vi "09_another_example.vi"() -> ()   [LabVIEW 2018, in "LV2Julia_examples.lvlib"]
uses:
  LV2Julia_examples.lvlib
  LV2Julia_core/VIs/Server or client state.ctl
  LV2Julia_core/VIs/detailed error info.ctl
  LV2Julia_core/VIs/StackFrame.ctl
  simple examples functions.ctl
  LV2Julia_core/VIs/Commands.ctl
  63b50369-e720-4ad2-b7fe-b63add1d9180.vi
  edf81fa3-46bf-427f-9605-85b461656974.vi
  29886417-d43f-41fb-9c0c-469db3f8c96d.vi
  3fe35f36-217a-40a5-a789-8326c52a1f5c.vi
  8d86b089-302c-401c-ae82-d9ebdf0ff266.vi
  35a44a82-786b-41ea-be73-9a4468e4df9d.vi
  a43e0667-dcfc-466a-94c9-f7da2d4fd36f.vi
  <vilib>/Utility/High Resolution Relative Seconds.vi
  edf81fa3-46bf-427f-9605-85b461656974.vi/ed560bc2-c7a5-459b-9b5d-c09f4150f87a.vi
  29886417-d43f-41fb-9c0c-469db3f8c96d.vi/351cf3e2-3c27-4899-8ca9-cb74734acfc8.vi
  3fe35f36-217a-40a5-a789-8326c52a1f5c.vi/3d491d8d-1e21-4aec-9a68-d7bbb94dfa6b.vi
  35a44a82-786b-41ea-be73-9a4468e4df9d.vi/70e9cb77-3a98-433e-ba66-4dcec83fe426.vi
  35a44a82-786b-41ea-be73-9a4468e4df9d.vi/c7757579-5117-4a7e-a803-a4a1d792155f.vi
  edf81fa3-46bf-427f-9605-85b461656974.vi/ed560bc2-c7a5-459b-9b5d-c09f4150f87a.vi/acba61d8-f5e3-4002-bc70-34f15e56434e.vi
  29886417-d43f-41fb-9c0c-469db3f8c96d.vi/351cf3e2-3c27-4899-8ca9-cb74734acfc8.vi/26bd0686-ce58-4dc2-9cfb-ec11559fc1fa.vi
  29886417-d43f-41fb-9c0c-469db3f8c96d.vi/351cf3e2-3c27-4899-8ca9-cb74734acfc8.vi/31514e23-2cd5-4295-b47a-a1ad325a4df0.vi
  29886417-d43f-41fb-9c0c-469db3f8c96d.vi/351cf3e2-3c27-4899-8ca9-cb74734acfc8.vi/3d30d75b-34ec-4e52-a519-b86950648cc6.vi
  3fe35f36-217a-40a5-a789-8326c52a1f5c.vi/3d491d8d-1e21-4aec-9a68-d7bbb94dfa6b.vi/5fb8a6ea-f43c-4306-9aef-f7be33a28f7f.vi
  3fe35f36-217a-40a5-a789-8326c52a1f5c.vi/3d491d8d-1e21-4aec-9a68-d7bbb94dfa6b.vi/dfcd26d4-3f06-4489-82d4-95ea86395353.vi
  3fe35f36-217a-40a5-a789-8326c52a1f5c.vi/3d491d8d-1e21-4aec-9a68-d7bbb94dfa6b.vi/9b688aa8-4353-46ee-ad38-c3c6feb92501.vi
  35a44a82-786b-41ea-be73-9a4468e4df9d.vi/70e9cb77-3a98-433e-ba66-4dcec83fe426.vi/97f29e4c-2cc7-47ea-9755-65b879169f6c.vi
  35a44a82-786b-41ea-be73-9a4468e4df9d.vi/70e9cb77-3a98-433e-ba66-4dcec83fe426.vi/9acd3ce5-a096-44ea-970d-7ed2f22121f9.vi
  edf81fa3-46bf-427f-9605-85b461656974.vi/ed560bc2-c7a5-459b-9b5d-c09f4150f87a.vi/acba61d8-f5e3-4002-bc70-34f15e56434e.vi/0e04b98d-ee84-41a3-96e8-138e19c14a1d.vi
  35a44a82-786b-41ea-be73-9a4468e4df9d.vi/70e9cb77-3a98-433e-ba66-4dcec83fe426.vi/97f29e4c-2cc7-47ea-9755-65b879169f6c.vi/a4bd5a91-b8fb-45c2-8725-513a162f3679.vi
  LV2Julia_core/VIs/jl-scripts path.vi
  LV2Julia_core/VIs/check ID validity.vi
  LV2Julia_core/VIs/bindata_descr to JSON.vi
  LV2Julia_core/VIs/check cluster field names.vi
  LV2Julia_core/VIs/concat JSON.vi
  LV2Julia_core/VIs/build request.vi
  LV2Julia_core/VIs/Parse server response.vi
  LV2Julia_core/VIs/log jl exceptions.vi
  <vilib>/Utility/error.llb/Error Cluster From Error Code.vi
  LV2Julia_core/LV2Julia_core.lvlib
  <vilib>/measure/NI_MABase.lvlib
panel:
  out "ZMQ timeout":bool
  out "Julia script file path":path
  out "temporary script path":path
  out "Jl Server state":T1
  in  "execution control pages":enum32{"Start", "go - test"}(tab)
  in  "go":bool caption="go (Julia Server started externally)"
  in  "Start with Julia":bool caption="Start Julia Server and go"
  in  "ZMQ endpoint":string="tcp://127.0.0.1:5555"
  in  "p":dbl=1.0
  in  "fn":T2 caption="select function at Server" items=["arr_amplitude", "arr_length", "arr_mean", "arr_median", "arr_rms", "vec_amplify", "vec_attenuate", "vec_power"]
  in  "trim @ begin":dbl min=0.0 max=100.0 step=1.0 format="%#.1f%%"
  in  "trim @ end":dbl min=0.0 max=200.0 step=1.0 format="%#.1f%%"
  in  "Group":T3(tab)
  out "Server response":dbl
  out "data received plot":dbl[](graph)
  out "data received":dbl[](array[numeric]) format="%.3f"
  out "RMS":dbl
  out "detailed error info":T4
  out "current error":errorcluster
  out "final error":errorcluster
  out "short err code":u8
  in  "tones":T6(array[cluster])=[{"frequency"=10.0, "amplitude"=1.0, "phase"=0.0}, {"frequency"=20.0, "amplitude"=0.1, "phase"=0.0}] {"phase" format="%.2p"; "amplitude" format="%0.2p"; "frequency" format="%0.2p"}
  in  "noise (rms)":dbl=0.1 format="%.2p"
  in  "offset":dbl format="%.2p"
  in  "sampling info":cluster{"Fs":dbl, "#s":dbl}={"Fs"=1000.0, "#s"=1000.0} {"Fs" format="%.2p"}
  in  "next":bool
  out "data sent to server":dbl[](graph)
  out "data sent":dbl[](array[numeric]) format="%.3f"
  out "function name":string
  in  "stop this VI only":bool
  in  "stop both this VI and Julia Server":bool
  out "call duration (ms)":dbl format="%#.2f"
  # "tcp://127.0.0.1:5555 \nfor local Julia Server\n\nFor a Julia Server running on a separate computer,  you probably must use an IPv4 address in numeric form (not a DNS name) - see https://stackoverflow.com/questions/6024003/why-doesnt-zeromq-work-on-localhost.\n\nThis control only used if Julia Server is not being started by this VI."
  # "generate sample array"
  # "function and parameter"
  # "enter a negative or a large positive value to cause an exception"
  # "data returned by server"
  # "data sent to server"
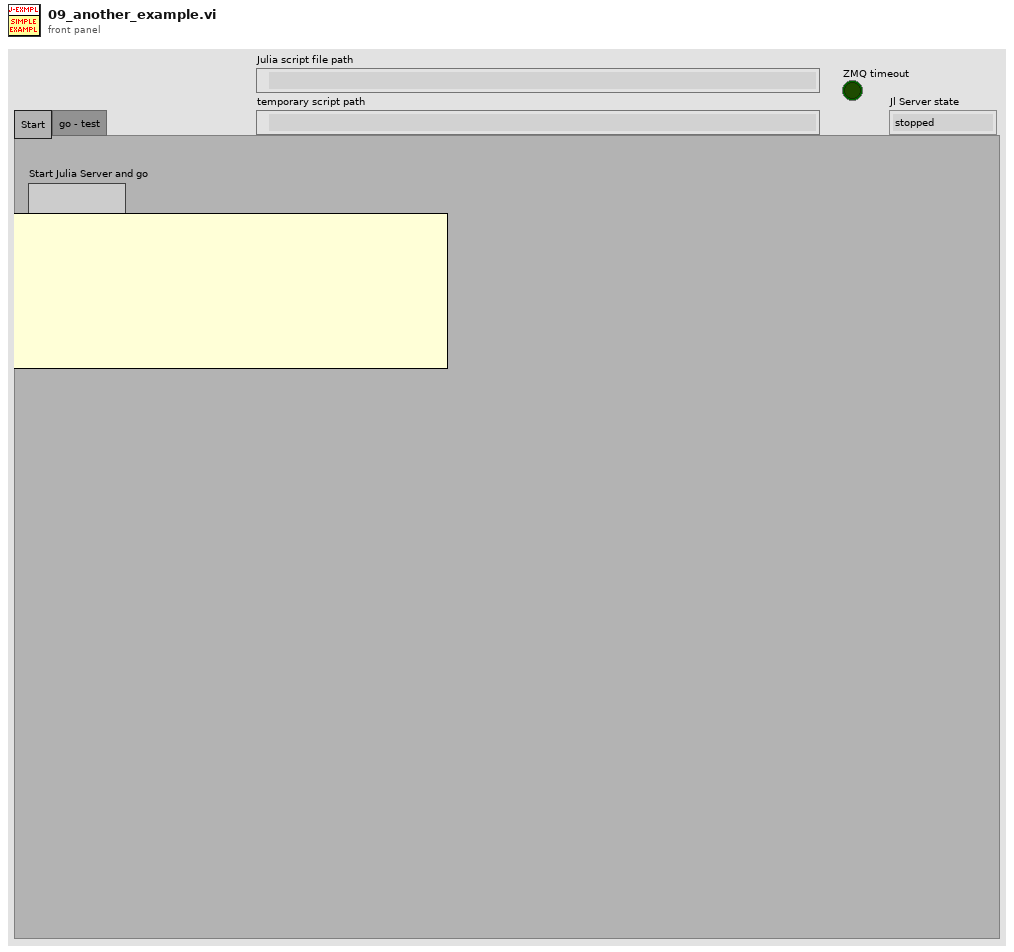
[diagram p1: front panel]
types:
  T1 = typedef "LV2Julia_core.lvlib/Server or client state.ctl" = enum16{"stopped", "running", "unknown"}
  T2 = typedef "LV2Julia_examples.lvlib/simple examples functions.ctl" = u16
  T3 = enum32{"fns returning scalar", "fns returning vector", "error"}
  T4 = typedef "LV2Julia_core.lvlib/detailed error info.ctl" = cluster{"exception_or_info":string, "trace":T5[]}
  T5 = typedef "LV2Julia_core.lvlib/StackFrame.ctl" = cluster{"frame_summary":string, "func":string, "linfo":string, "file":string, "line":i32, "pointer":u64, "from_c":bool, "inlined":bool}
  T6 = cluster{"frequency":dbl, "amplitude":dbl, "phase":dbl}[]
  T7 = typedef "LV2Julia_core.lvlib/Commands.ctl" = enum16{"Start Jl-server & Init LV-client", "Send request & Get response ", "Stop Jl-server & Cleanup LV-client", "Cleanup LV-client", "Start Jl-server", "Stop Jl-server", "Init LV-Client", "Cleanup LV-Client", "(not allowed)", "Set LV Client state", "Set Jl Server state", "set ZMQ timeout", "read ZMQ timeout", "read-out state"}
  T8 = enum8{"Enabled", "Disabled", "Disabled and Grayed Out"}
  T9 = typedef "LV2Julia_core.lvlib/Bindata&description.ctl" = cluster{"bindata_descr":T10[], "bindata":u8[]}
  T10 = typedef "LV2Julia_core.lvlib/Bindata description.ctl" = cluster{"nofbytes":i32, "numtype":string, "start":i32, "arrdims":i32[], "kwarg_name":string, "category":string}
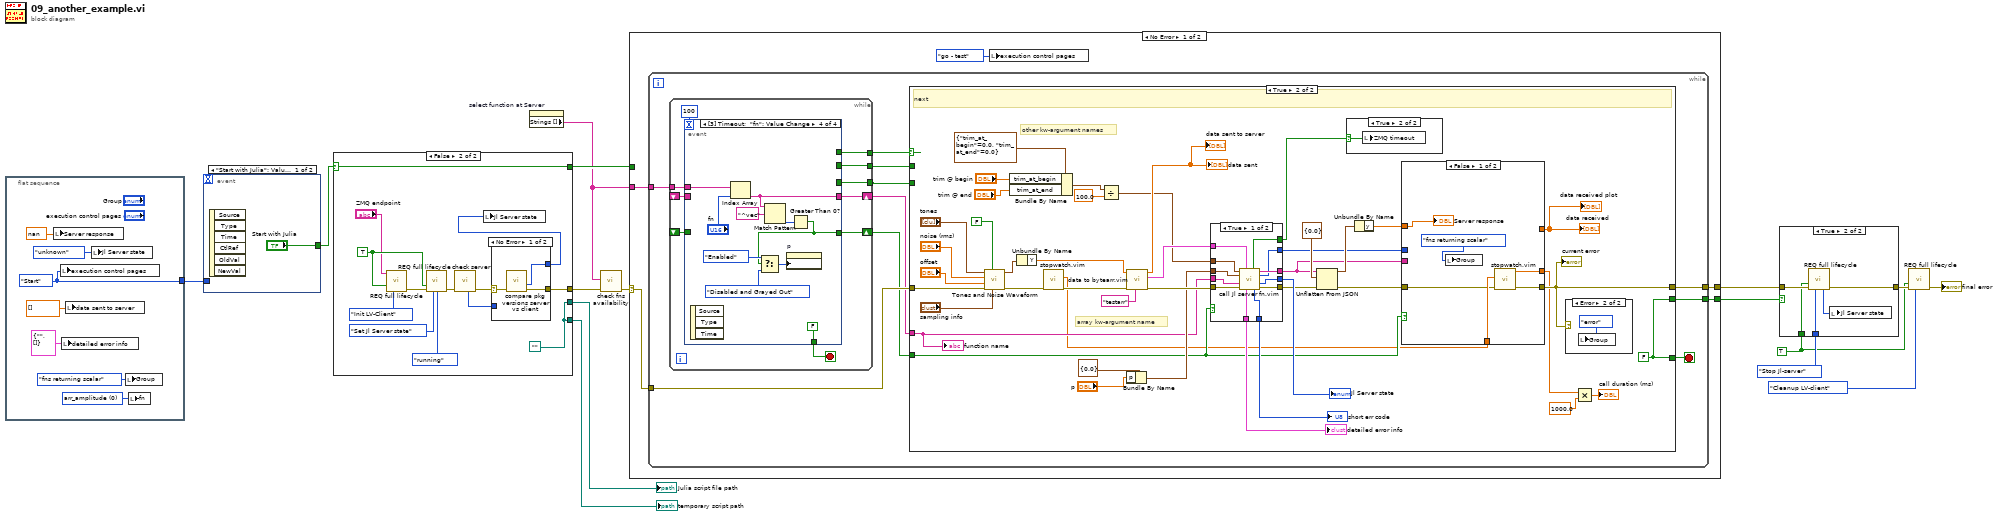
[diagram p0: block diagram]
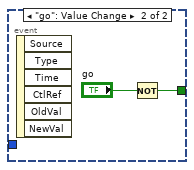
[diagram p2: hidden frame]
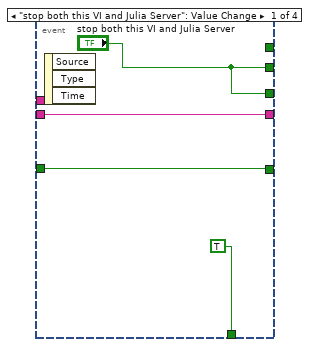
[diagram p3: hidden frame]
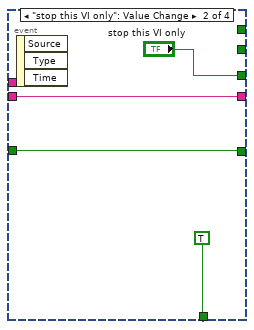
[diagram p4: hidden frame]
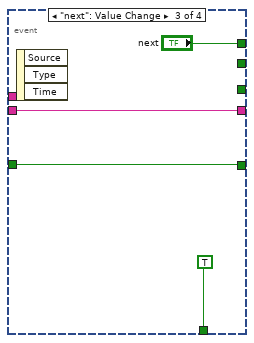
[diagram p5: hidden frame]
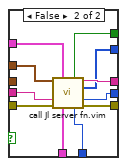
[diagram p7: hidden frame]
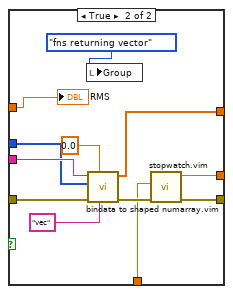
[diagram p9: hidden frame]
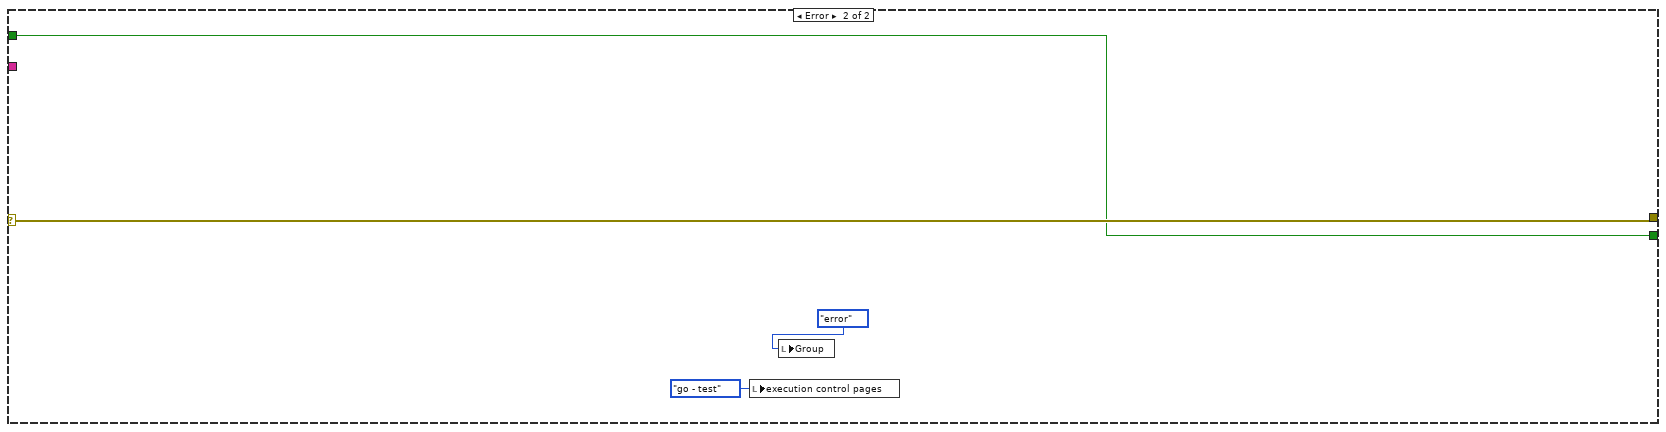
[diagram p11: hidden frame]
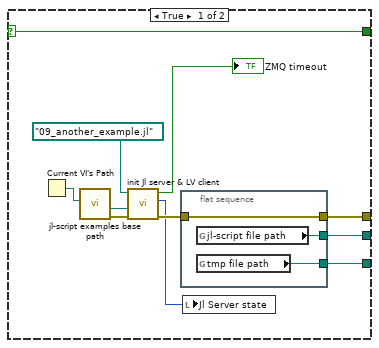
[diagram p12: hidden frame]
diagram:
  w10 = TRUE ("Force command")
  n1 = flat-sequence {
    tunnel: [w22] -> w6
    frame #0 {
      w16 = T2 0 items=["arr_amplitude", "arr_length", "arr_mean", "arr_median", "arr_rms", "vec_amplify", "vec_attenuate", "vec_power"] ("fn")
      w22 = enum32{"Start", "go - test", "finish"}."Start" ("execution control pages")
      n2 = local write "Server response"(nan ("Server response")) -> ()
      n3 = local write "execution control pages"(w22) -> ()
      n4 = local write "detailed error info"(T4 {"exception_or_info"="", "trace"=[]} ("detailed error info")) -> ()
      n5 = local write "data sent to server"(dbl[] []) -> ()
      n6 = local write "Jl Server state"(Server_or_client_state."unknown" ("Jl Server state out")) -> ()
      n7 = local write "Group"(T3."fns returning scalar" ("Group")) -> ()
      n8 = local write "fn"(w16) -> ()
    }
  }
  n9 = event shown="[0] \"Start with Julia\": Value Change" {
    selector: _ -> [_ _]
    dyn-events: _ -> [_ _]
    timeout: _ -> [_ _]
    tunnel: ["Start with Julia" w24] -> w8
    tunnel: w6 -> [_ _]
    event "Start with Julia": Value Change {
      n10 = event-data() -> ()  [unwired: 1 in, 6 out]
    }
    event "go": Value Change {
      n11 = event-data() -> ()  [unwired: 1 in, 6 out]
      n12 = Not(x="go") -> (.not. x?=w24:bool)
    }
  }
  n13 = case shown="False" w8 {
    selector: w8 -> [w36 w48]
    tunnel: [w35 w42] -> w5
    tunnel: [w36 w48] -> w7
    tunnel: [w34 w45] -> w1
    tunnel: [w33 w45] -> w2
    frame True {
      n14 = Current VI's Path() -> (path=w28:path)
      n15 = call "jl-script examples base path.vi"("calling example VI path"=w28) -> ("error out"=w27:errorcluster, "jl-script-examples base path"=w26:path)  [unwired: 9 in]
      n16 = call "init Jl server & LV client.vi"("error in (no error)"=w27, "Base path (not a path)"=w26, "Julia user functions script"=path "09_another_example.jl") -> ("error out"=w30:errorcluster, "Jl Server state out"=w29:T1, "timeout?"=→"ZMQ timeout":bool)  [unwired: 6 in]
      n17 = flat-sequence {
        tunnel: [w39] -> w35
        tunnel: w30 -> [w39]
        tunnel: [w38] -> w34
        tunnel: [w37] -> w33
        frame #0 {
          n18 = global read "jl-scripts path.vi" "jl-script file path"() -> (w38:path)
          n19 = global read "jl-scripts path.vi" "tmp file path"() -> (w37:path)
        }
      }
      n20 = local write "Jl Server state"(w29) -> ()
    }
    frame False {
      w45 = path ""
      w50 = TRUE ("Force command")
      n21 = call "REQ full lifecycle.vi"("ZMQ endpoint"="ZMQ endpoint", "Force command"=w50, "command"=Commands."Init LV-Client") -> ("error out"=w47:errorcluster)  [unwired: 6 in, 6 out]
      n22 = call "REQ full lifecycle.vi"("Force command"=w50, "error in"=w47, "command"=Commands."Set Jl Server state", "Jl Server state in"=Server_or_client_state."running") -> ("error out"=w46:errorcluster)  [unwired: 5 in, 6 out]
      n23 = call "check server.vi"("error in"=w46) -> ("error out"=w43:errorcluster, "Jl Server state out"=w41:T1)  [unwired: 6 in, 3 out]
      n24 = case shown="No Error" w43 {
        selector: w43 -> [w55 w57]
        tunnel: [w54 w57] -> w42
        tunnel: [w53 w56] -> w40
        tunnel: w41 -> [_ w56]
        frame No Error {
          n25 = call "compare pkg versions server vs client.vi"("error in (no error)"=w55) -> ("error out"=w54:errorcluster, "Jl Server state out"=w53:T1)  [unwired: 4 in, 5 out]
        }
        frame Error {
        }
      }
      n26 = local write "Jl Server state"(w40) -> ()
    }
  }
  "temporary script path" <- w2
  "Julia script file path" <- w1
  n27 = property on="select function at Server" class="Ring (strict)"() -> ("Strings []"=w3:string[])  [unwired: 2 in, 2 out]
  n28 = call "check fns availability.vi"("error in (no error)"=w5, "fns list is"=w3) -> ("error out"=w4:errorcluster)  [unwired: 3 in, 6 out]
  n29 = case shown="No Error" w4 {
    selector: w4 -> [w61 w197]
    tunnel: [w62 w197] -> w15
    tunnel: [w60 w196] -> w9
    tunnel: w3 -> [w59 _]
    tunnel: w7 -> [_ w196]
    frame No Error {
      n30 = while {
        tunnel: w61 -> [w71]
        tunnel: [w72] -> w62
        tunnel: [w68] -> w60
        tunnel: w59 -> [w66]
        stop <- w69 stop-if-true
        n31 = while {
          tunnel: [w82] -> w70
          tunnel: [w81] -> w67
          tunnel: w66 -> [w78]
          shift-right: [w77] -> w65
          shift-left: _ -> [w74]
          shift-right: [w76] -> w64
          shift-left: _ -> [w75]
          tunnel: [w73] -> w63
          stop <- w80 stop-if-true
          n32 = event shown="[3] Timeout;  \"fn\": Value Change" {
            selector: _ -> [_ _ _ _]
            dyn-events: _ -> [_ _ _ _]
            timeout: 100 -> [_ _ _ _]
            tunnel: ["stop both this VI and Julia Server" _ _ _] -> w81
            tunnel: [_ _ "next" _] -> w82
            tunnel: [TRUE TRUE TRUE FALSE] -> w80
            tunnel: w78 -> [_ _ _ w98]
            tunnel: [w84 w88 w92 w97] -> w77
            tunnel: [w85 w89 w91 w96] -> w76
            tunnel: w75 -> [w85 w89 w91 _]
            tunnel: w74 -> [w84 w88 w92 _]
            tunnel: ["stop both this VI and Julia Server" "stop this VI only" _ _] -> w73
            event "stop both this VI and Julia Server": Value Change {
              n33 = event-data() -> ()  [unwired: 1 in, 3 out]
            }
            event "stop this VI only": Value Change {
              n34 = event-data() -> ()  [unwired: 1 in, 3 out]
            }
            event "next": Value Change {
              n35 = event-data() -> ()  [unwired: 1 in, 3 out]
            }
            event Timeout; Value Change {
              n36 = event-data() -> ()  [unwired: 1 in, 3 out]
              n37 = Index Array(array=w98, index="fn") -> (element=w96:string)
              n38 = Match Pattern(string=w96, regular expression="^vec") -> (offset past match=w102:i32)  [unwired: 1 in, 3 out]
              n39 = Greater Than 0?(x=w102) -> (x > 0?=w97:bool)
              n40 = Select(t=T8."Enabled" ("Disabled"), s=w97, f=T8."Disabled and Grayed Out" ("Disabled")) -> (s? t:f=w104:T8)
              n41 = property on="p" class="DigNum (strict)"("DisabledEnum"=w104) -> ()  [unwired: 2 in, 2 out]
            }
          }
        }
        n42 = case shown="True" w70 {
          tunnel: [w107 w132] -> w72
          tunnel: w71 -> [w107 w137]
          tunnel: [w106 w136] -> w69
          tunnel: w63 -> [w106 _]
          tunnel: [w105 w136] -> w68
          tunnel: w67 -> [w105 _]
          tunnel: w65 -> [_ w119]
          tunnel: w64 -> [_ w121]
          frame False {
            # "stop"
          }
          frame True {
            w136 = FALSE ("stop this VI only")
            # "other kw-argument names"
            # "array kw-argument name"
            # "next"
            n43 = call <vilib>:"Tones and Noise Waveform.vi"("sampling info"="sampling info", "reset signal"=FALSE, "error in (no error)"=w137, "offset"="offset", "noise (rms)"="noise (rms)", "tones"="tones") -> ("error out"=w111:errorcluster, "signal out"=w143:waveform(dbl))  [unwired: 4 in]
            n44 = Bundle By Name(cluster=cluster{"trim_at_begin":dbl, "trim_at_end":dbl} {"trim_at_begin"=0.0, "trim_at_end"=0.0}, "trim_at_begin"="trim @ begin", "trim_at_end"="trim @ end") -> (w116:cluster{"trim_at_begin":dbl, "trim_at_end":dbl})
            n45 = Unbundle By Name(w143) -> ("Y"=w138:dbl[])
            n46 = call "stopwatch.vim"("anything in"=w111) -> ("copy of anything out"=w110:errorcluster, "current timepoint"=w109:dbl)  [unwired: 8 in, 1 out]
            n47 = Divide(x=w116, y=100.0 ("trim @ end")) -> (x/y=w117:cluster{"trim_at_begin":dbl, "trim_at_end":dbl})
            n48 = call "data to bytearr.vim"("kwarg_name"="testarr", "error in (no error)"=w110, "data in"=w138) -> ("error out"=w130:errorcluster, "Bindata & descr out"=w123:T9, "flattened data out"=→"data sent" →"data sent to server":dbl[])  [unwired: 6 in]
            n49 = Bundle By Name(cluster=cluster{"p":dbl} {"p"=0.0}, "p"="p") -> (w122:cluster{"p":dbl})
            n50 = case shown="True" w119 {
              tunnel: w130 -> [w162 w173]
              tunnel: [w161 w172] -> w129
              tunnel: [w160 w171] -> w128
              tunnel: [w159 w170] -> w127
              tunnel: [w158 w169] -> w126
              tunnel: [w157 w168] -> w125
              tunnel: [w156 w167] -> w124
              tunnel: w123 -> [w155 w166]
              tunnel: w117 -> [w154 w165]
              tunnel: w122 -> [w153 _]
              tunnel: w121 -> [w152 w164]
              tunnel: [w151 w163] -> w120
              frame True {
                n51 = call "call Jl server fn.vim"("Arguments 1"=w154, "Bindata & descr in"=w155, "Arguments 2"=w153, "fun2call"=w152, "error in (no error)"=w162) -> ("timeout?"=w156:bool, "JSON received"=w158:string, "binary data received"=w157:u8[], "Jl Server state out"=w160:T1, "detailed error info"=w161:T4, "return code"=w151:u8, "error out"=w159:errorcluster)  [unwired: 4 in]
              }
              frame False {
                n52 = call "call Jl server fn.vim"("Arguments 1"=w165, "Bindata & descr in"=w166, "fun2call"=w164, "error in (no error)"=w173) -> ("timeout?"=w167:bool, "JSON received"=w169:string, "binary data received"=w168:u8[], "Jl Server state out"=w171:T1, "detailed error info"=w172:T4, "return code"=w163:u8, "error out"=w170:errorcluster)  [unwired: 5 in]
              }
            }
            "short err code" <- w120
            "Jl Server state" <- w128
            "detailed error info" <- w129
            n53 = Unflatten From JSON(JSON string=w126, type and defaults=cluster{"y":dbl} {"y"=0.0} ("parsed response"), error in (no error)=w127) -> (value=w149:cluster{"y":dbl}, error out=w133:errorcluster)  [unwired: 4 in]
            n54 = case shown="True" w124 {
              selector: w124 -> [_ w174]
              frame False {
              }
              frame True {
                n55 = local write "ZMQ timeout"(w174) -> ()
              }
            }
            n56 = Unbundle By Name(w149) -> ("y"=w131:dbl)
            n57 = case shown="False" w119 {
              tunnel: w133 -> [w175 w191]
              tunnel: [w176 w183] -> w132
              tunnel: w125 -> [_ w186]
              tunnel: w126 -> [_ w187]
              tunnel: w131 -> [w179 w189]
              tunnel: [w177 w181] -> w108
              tunnel: [_ w185] -> w112
              tunnel: w109 -> [w178 w182]
              frame False {
                n58 = local write "Group"(T3."fns returning scalar" ("Group")) -> ()
                n59 = call "stopwatch.vim"("anything in"=w175, "prev timepoint (0)"=w178) -> ("copy of anything out"=w176:errorcluster, "delta t (s)"=w177:dbl)  [unwired: 7 in, 1 out]
                "Server response" <- w179
              }
              frame True {
                n60 = local write "Group"(T3."fns returning vector" ("Group")) -> ()
                n61 = call "bindata to shaped numarray.vim"("name"="vec" ("kwarg_name"), "element type"=0.0 ("data type"), "error in (no error)"=w191, "binary data"=w186, "JSON in"=w187) -> ("error out"=w184:errorcluster, "numarray 1D"=w185:dbl[])  [unwired: 3 in, 2 out]
                n62 = call "stopwatch.vim"("anything in"=w184, "prev timepoint (0)"=w182) -> ("copy of anything out"=w183:errorcluster, "delta t (s)"=w181:dbl)  [unwired: 7 in, 1 out]
                "RMS" <- w189
              }
            }
            "current error" <- w132
            "data received plot" <- w112
            "data received" <- w112
            n63 = case shown="Error" w132 {
              frame No Error {
              }
              frame Error {
                n64 = local write "Group"(T3."error" ("Group")) -> ()
              }
            }
            n65 = Multiply(x=w108, y=1000.0) -> (x*y=→"call duration (ms)":dbl)
            "function name" <- w121
          }
        }
      }
      n66 = local write "execution control pages"(enum32{"Start", "go - test", "finish"}."go - test" ("execution control pages")) -> ()
    }
    frame Error {
      n67 = local write "execution control pages"(enum32{"Start", "go - test", "finish"}."go - test" ("execution control pages")) -> ()
      n68 = local write "Group"(T3."error" ("Group")) -> ()
    }
  }
  n69 = case shown="True" w9 {
    tunnel: w15 -> [w198 w203]
    tunnel: Commands."Stop Jl-server" ("command") -> [_ w202]
    tunnel: [w198 w201] -> w13
    tunnel: w10 -> [_ w200]
    frame False {
    }
    frame True {
      n70 = call "REQ full lifecycle.vi"("Force command"=w200, "error in"=w203, "command"=w202) -> ("Jl Server state out"=w199:T1, "error out"=w201:errorcluster)  [unwired: 6 in, 5 out]
      n71 = local write "Jl Server state"(w199) -> ()
    }
  }
  n72 = call "REQ full lifecycle.vi"("Force command"=w10, "error in"=w13, "command"=Commands."Cleanup LV-client") -> ("error out"=→"final error":errorcluster)  [unwired: 6 in, 6 out]
